vi "TRIG_CHAN_ROUT_INP.vi"(0 "VISA IN":refnum<visa-resource-name>, 1 "Input":string(combo)="MAIN", 5 "error in":errorcluster, 7 "Channel":i32) -> (14 "VISA Out":refnum<visa-resource-name>, 19 "error out":errorcluster)   [LabVIEW 2018, in "PNA-X.lvlib"]
doc: "TRIGger:CHANnel<ch>:ROUTe:INPut <char> \n(Read-Write) Specifies the connector to use for the external trigger input.(Similar to \nCONTROL:SIGNal <conn>) \nParameters \n<ch> Any existing channel number. If unspecified, value is set to 1. \n<char> Choose from: \nMAIN - meas trig ready \nMATH - material handler \nAUXT - auxio (PNA-L and E836xB ONLY) \nExamples TRIG:CHAN:ROUT:INP MAIN \ntrigger:channel2:route:input main \nQuery Syntax TRIGger:CHANnel<ch>:ROUTe:INPut? \nReturn Type Character \nDefault"
uses:
  PNA-X.lvlib
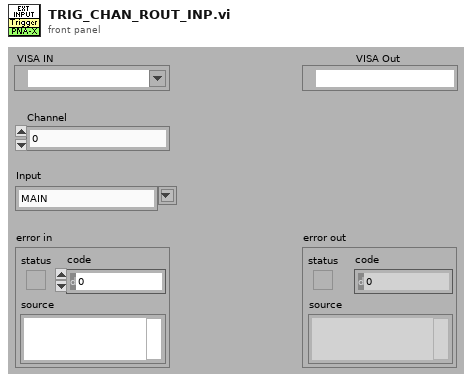
[diagram p1: front panel]
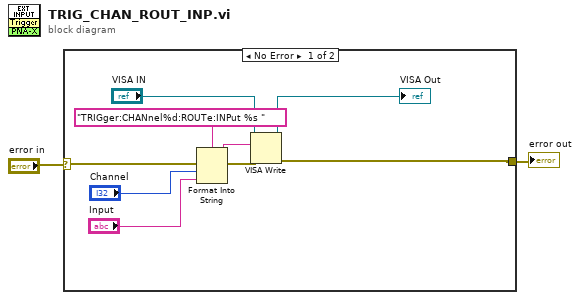
[diagram p0: block diagram]
diagram:
  n1 = case shown="No Error" "error in" {
    selector: "error in" -> [w11 w12]
    tunnel: [w6 w12] -> w1
    frame No Error {
      n2 = Format Into String(format string="TRIGger:CHANnel%d:ROUTe:INPut %s " ("Cmdline"), error in=w11, "Channel", "Input") -> (resulting string=w9:string, error out=w10:errorcluster)  [unwired: 1 in]
      n3 = VISA Write(VISA resource name="VISA IN", write buffer=w9, error in (no error)=w10) -> (VISA resource name out=→"VISA Out":refnum<visa-resource-name>, error out=w6:errorcluster)  [unwired: 1 out]
    }
    frame Error {
    }
  }
  "error out" <- w1
